vi "Read Value.vi"(8 "error in (no error)":errorcluster, 11 "sfixed32 in":refnum<class "sfixed32.lvclass">) -> (0 "error out":errorcluster, 2 "Value":i32, 3 "sfixed32 out":refnum<class "sfixed32.lvclass">)   [LabVIEW 2020, in "Protobuf RAW.lvlib" / "sfixed32.lvclass"]
uses:
  sfixed32.lvclass
  sfixed32.lvclass/sfixed32.ctl
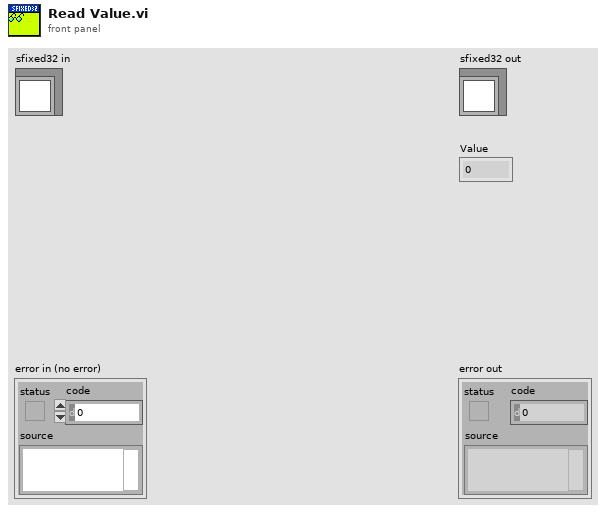
[diagram p1: front panel]
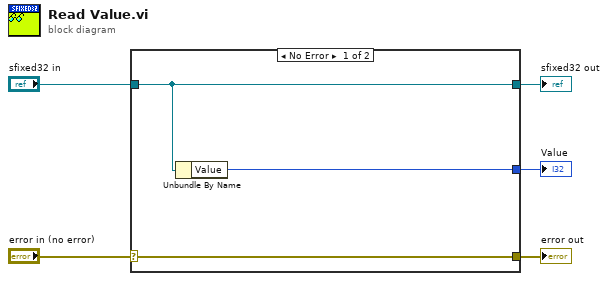
[diagram p0: block diagram]
diagram:
  n1 = case shown="No Error" "error in (no error)" {
    selector: "error in (no error)" -> [w8 w9]
    tunnel: [w8 w9] -> w4
    tunnel: [w7 w10] -> w2
    tunnel: "sfixed32 in" -> [w7 w10]
    tunnel: [w6 _] -> w1
    frame No Error {
      n2 = Unbundle By Name(w7) -> ("Value"=w6:i32)
    }
    frame Error {
    }
  }
  "error out" <- w4
  "sfixed32 out" <- w2
  "Value" <- w1
